vi "Write Power Supply.lvclass.vi"(10 "Power Supply lvclasses":refnum<class "Power Supply.lvclass">[](array[class]), 11 "Test Framework in":refnum<class "Test Framework.lvclass">) -> (3 "Test Framework out":refnum<class "Test Framework.lvclass">)   [LabVIEW 2020, in "Test Framework.lvclass"]
uses:
  Test Framework.lvclass
  Instruments/Power Supply/Power Supply.lvclass
  Test Framework.lvclass/Test Framework.ctl
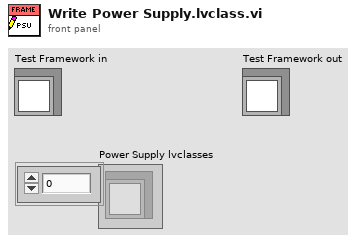
[diagram p1: front panel]
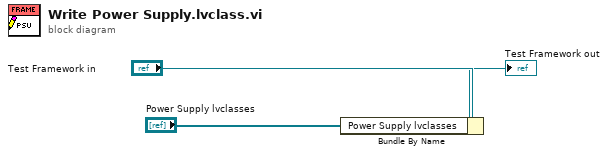
[diagram p0: block diagram]
diagram:
  n1 = Bundle By Name(cluster="Test Framework in", "Power Supply lvclasses"="Power Supply lvclasses") -> (→"Test Framework out":refnum<class "Test Framework.lvclass">)
